vi "GE 5565PIORC.Open.vi"(8 "error in (no error)":errorcluster, 11 "VISA resource name":refnum<visa-resource-name>) -> (0 "error out":errorcluster, 3 "GE 5565PIORC.lvclass":refnum<class "GE 5565PIORC.lvclass">)   [LabVIEW 2016, in "GE 5565PIORC.lvclass"]
doc: "Opens a new VISA session to the GE Reflective Memory card."
uses:
  GE 5565PIORC.lvclass
  GE 5565PIORC.lvclass/GE 5565PIORC.ctl
  Properties/Registers/GE 5565PIORC.Registers.Local Configuration.Read.vi
  Properties/Registers/GE 5565PIORC.Registers.Local Configuration.Read (U32).vi
  GE 5565PIORC.Registers.Read.vi
  GE 5565PIORC.Registers.Read (U32).vi
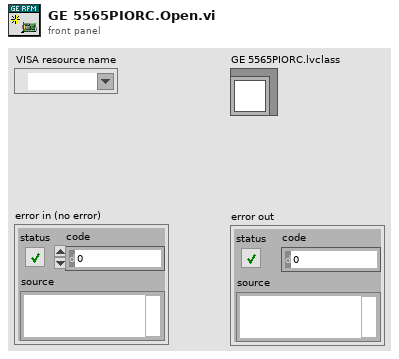
[diagram p1: front panel]
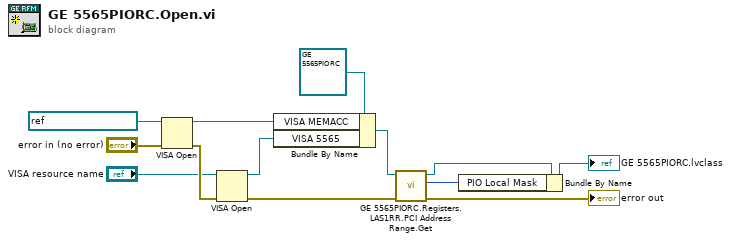
[diagram p0: block diagram]
diagram:
  n1 = VISA Open(error in (no error)="error in (no error)", VISA resource name=refnum<visa-resource-name> "PXI0::MEMACC") -> (VISA resource name=w6:refnum<visa-resource-name>, error out=w4:errorcluster)  [unwired: 3 in]
  n2 = VISA Open(error in (no error)=w4, VISA resource name="VISA resource name") -> (VISA resource name=w2:refnum<visa-resource-name>, error out=w3:errorcluster)  [unwired: 3 in]
  n3 = Bundle By Name(cluster=refnum<class "GE 5565PIORC.lvclass"> refnum ("GE 5565PIORC.lvclass"), "VISA MEMACC"=w6, "VISA 5565"=w2) -> (w10:refnum<class "GE 5565PIORC.lvclass">)
  n4 = call "GE 5565PIORC.Registers.LAS1RR.PCI Address Range.Get.vi"("error in (no error)"=w3, "GE 5565PIORC in"=w10) -> ("error out"=→"error out":errorcluster, "PCI Address Range"=w7:u32, "GE 5565PIORC out"=w8:refnum<class "GE 5565PIORC.lvclass">)  [unwired: 7 in]
  n5 = Bundle By Name(cluster=w8, "PIO Local Mask"=w7) -> (→"GE 5565PIORC.lvclass":refnum<class "GE 5565PIORC.lvclass">)
